vi "Concrete Type.vi"(8 "error in (no error)":errorcluster, 11 "Relation in":refnum<class "Relation.lvclass">) -> (0 "error out":errorcluster, 3 "Concrete Type":refnum<class "Type.lvclass">)   [LabVIEW 2020, in "Conditum.lvlib" / "Columns.lvlib" / "Relation.lvclass"]
uses:
  Relation.lvclass
  C:/dev/lv20CE/lv-conditum/Conditum/Columns/Type/Type.lvclass
  Type/Type.lvclass
  Relation.lvclass/Relation.ctl
  Entity/Entity.lvclass
  C:/dev/lv20CE/lv-conditum/Conditum/Columns/Relation/Relation.lvclass
  Entity Collection/Entity Collection.lvclass
  Relation Mapping.ctl
  Conditum.lvlib
  Relation Info.ctl
  Type/Definition.ctl
  Relation Definition.ctl
  C:/dev/lv20CE/lv-conditum/Conditum/Columns/Entity/Entity.lvclass
  C:/dev/lv20CE/lv-conditum/Conditum/Columns/Entity Collection/Entity Collection.lvclass
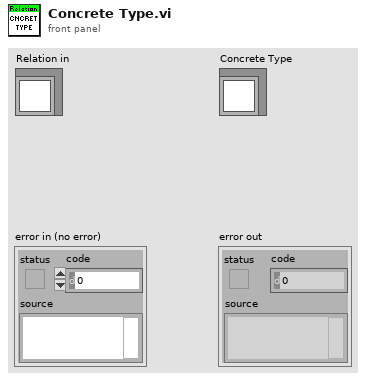
[diagram p1: front panel]
types:
  T1 = typedef "Conditum.lvlib/Columns.lvlib/Relation.lvclass/Relation Definition.ctl" = cluster{"Type":T2, "Relation":T3}
  T2 = typedef "Conditum.lvlib/Columns.lvlib/Type.lvclass/Definition.ctl" = cluster{"Name":string, "Nullable":bool, "Default NULL":bool}
  T3 = typedef "Conditum.lvlib/Relation Info.ctl" = cluster{"Mapping":T4, "Related To":string, "Reversed By":string}
  T4 = typedef "Conditum.lvlib/Relation Mapping.ctl" = enum16{"OneToOne", "OneToMany", "ManyToOne", "ManyToMany"}
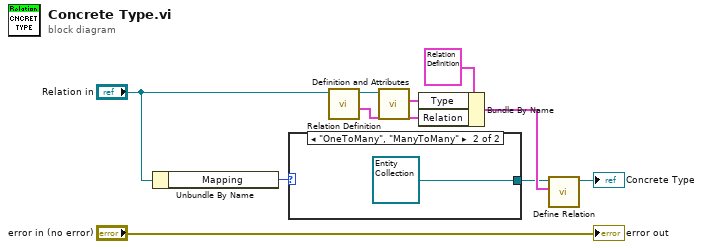
[diagram p0: block diagram]
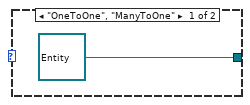
[diagram p2: hidden frame]
diagram:
  n1 = Unbundle By Name("Relation in") -> ("Mapping"=w10:T4)
  n2 = case shown="\"OneToMany\", \"ManyToMany\"" w10 {
    tunnel: [refnum<class "Entity.lvclass"> refnum ("Conditum:Columns:Entity.lvclass") refnum<class "Entity Collection.lvclass"> refnum ("Conditum:Columns:Entity Collection.lvclass")] -> w3
    frame "OneToOne", "ManyToOne" {
    }
    frame "OneToMany", "ManyToMany" {
    }
  }
  n3 = call "Relation Definition.vi"("Relation in"="Relation in") -> ("Relation Definition"=w6:T3, "Relation out"=w8:refnum<class "Relation.lvclass">)  [unwired: 8 in, 1 out]
  n4 = call "Definition and Attributes.vi"("Type in"=w8) -> ("Definition"=w7:T2)  [unwired: 8 in, 2 out]
  n5 = Bundle By Name(cluster=T1 {"Type"={"Name"="", "Nullable"=FALSE, "Default NULL"=FALSE}, "Relation"={"Mapping"=enum."OneToMany", "Related To"="", "Reversed By"=""}} ("Relation Definition"), "Type"=w7, "Relation"=w6) -> (w5:T1)
  n6 = call "Define Relation.vi"("Relation Definition"=w5, "Relation in"=w3) -> ("Relation out"=→"Concrete Type":refnum<class "Relation.lvclass">)  [unwired: 9 in]
  "error out" <- "error in (no error)"
